vi "Get Document Source.vi"(8 "Error In":errorcluster, 11 "object in":refnum<class "WebView.lvclass">) -> (0 "Error Out":errorcluster, 2 "Document Source":string, 3 "object out":refnum<class "WebView.lvclass">)   [LabVIEW 2024, in "WebView.lvclass"]
uses:
  <resource>/Framework/Providers/Open_GDS/ClassProviders/Provider_LvNativeClass/Templates/NativeBaseTemplate_4x4x4/NativeBaseTemplate_4x4x4.lvclass/NativeBaseTemplate_4x4x4.ctl
  WebView.lvclass
  WebView.lvclass/WebView.ctl
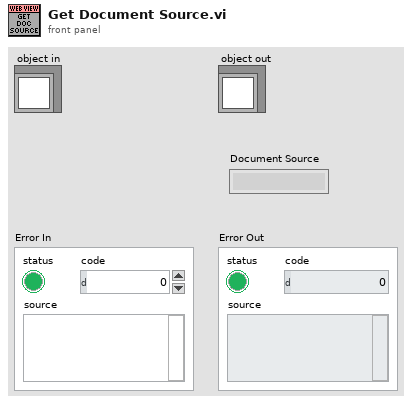
[diagram p1: front panel]
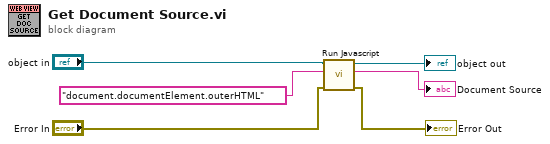
[diagram p0: block diagram]
diagram:
  n1 = call "Run Javascript.vi"("Error In"="Error In", "Javascript in"="document.documentElement.outerHTML" ("javaScript"), "object in"="object in") -> ("Error Out"=→"Error Out":errorcluster, "Result out"=→"Document Source":string, "object out"=→"object out":refnum<class "WebView.lvclass">)  [unwired: 6 in]
